vi "Read Real Allele.vi"(8 "error in (no error)":errorcluster, 11 "Real Gene in":refnum<class "Real Gene.lvclass">) -> (0 "error out":errorcluster, 2 "Real Allele":dbl, 3 "Real Gene out":refnum<class "Real Gene.lvclass">)   [LabVIEW 2016, in "Real Gene.lvclass"]
uses:
  Real Gene.lvclass
  Real Gene.lvclass/Real Gene.ctl
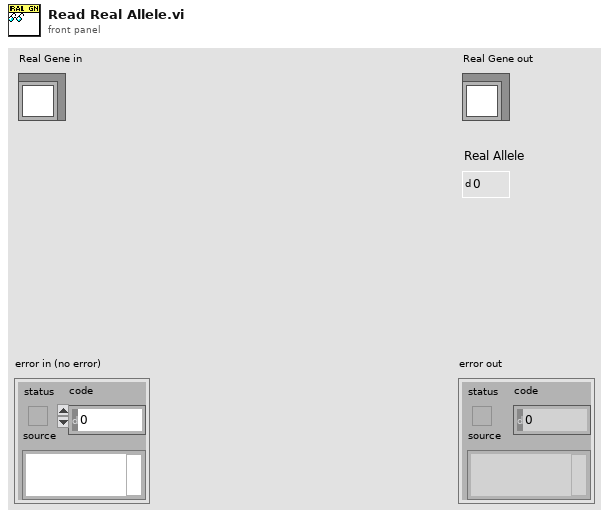
[diagram p1: front panel]
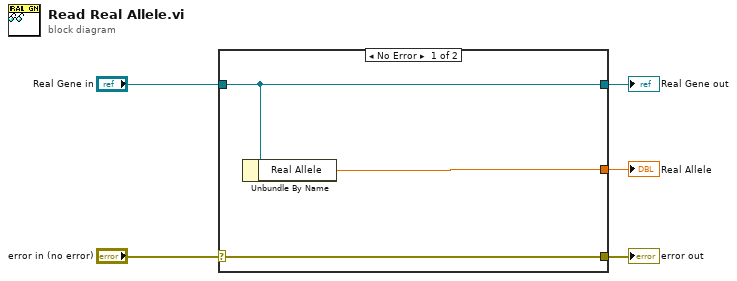
[diagram p0: block diagram]
diagram:
  n1 = case shown="No Error" "error in (no error)" {
    selector: "error in (no error)" -> [w8 w9]
    tunnel: [w8 w9] -> w4
    tunnel: [w7 w10] -> w2
    tunnel: "Real Gene in" -> [w7 w10]
    tunnel: [w6 _] -> w1
    frame No Error {
      n2 = Unbundle By Name(w7) -> ("Real Allele"=w6:dbl)
    }
    frame Error {
    }
  }
  "error out" <- w4
  "Real Gene out" <- w2
  "Real Allele" <- w1
